vi "Save Station Information.vi"(8 "error in (no error)":errorcluster, 10 "Station Info":T1, 11 "csv-formatter in":refnum<class "csv-formatter.lvclass">) -> (0 "error out":errorcluster, 3 "csv-formatter out":refnum<class "csv-formatter.lvclass">)   [LabVIEW 2015, in "csv-formatter.lvclass"]
doc: "This VI will save the DUT Information to the permanent report"
uses:
  csv-formatter.lvclass
  Report Information/Station Information.ctl
  csv-formatter.lvclass/csv-formatter.ctl
  Report Information/Report Information.lvclass
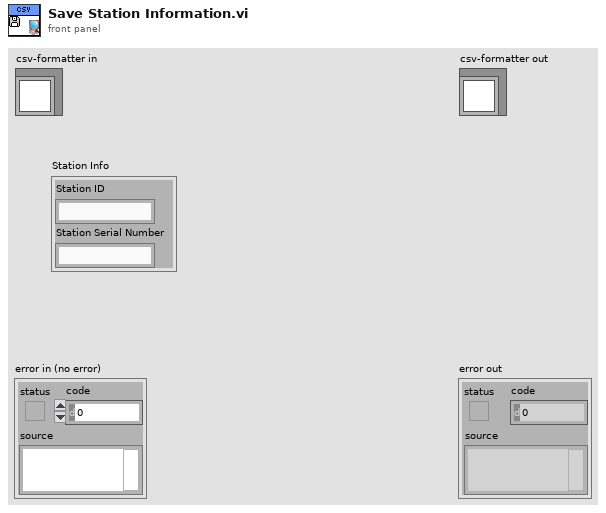
[diagram p1: front panel]
types:
  T1 = typedef "Report Information.lvclass/Station Information.ctl" = cluster{"Station ID":string, "Station Serial Number":string}
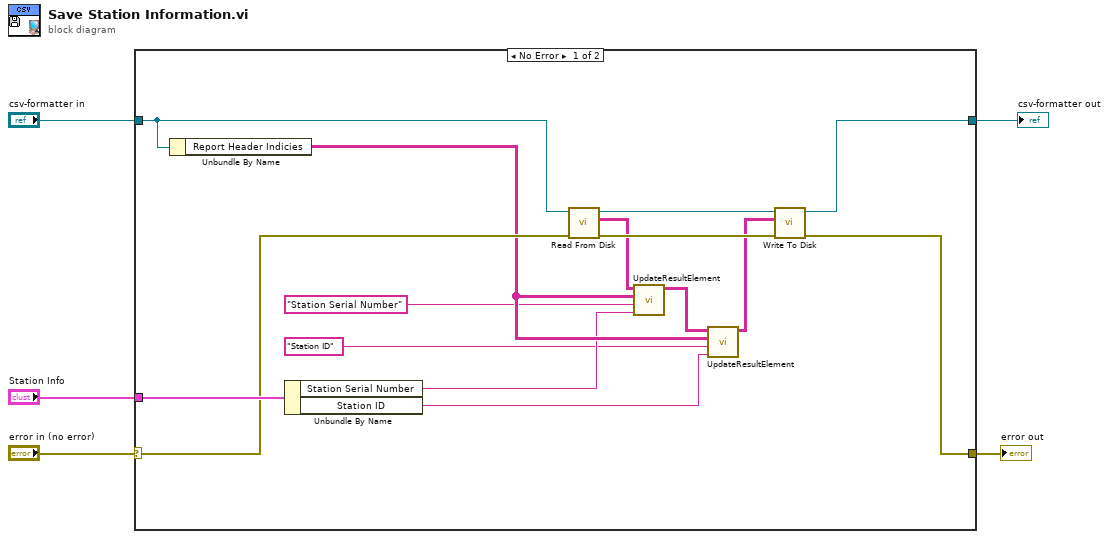
[diagram p0: block diagram]
diagram:
  n1 = case shown="No Error" "error in (no error)" {
    selector: "error in (no error)" -> [w19 w22]
    tunnel: "Station Info" -> [w20 _]
    tunnel: "csv-formatter in" -> [w14 w21]
    tunnel: [w17 w22] -> w2
    tunnel: [w15 w21] -> w1
    frame No Error {
      n2 = Unbundle By Name(w14) -> ("Report Header Indicies"=w10:string[][])
      n3 = Unbundle By Name(w20) -> ("Station Serial Number"=w8:string, "Station ID"=w6:string)
      n4 = call "Read From Disk.vi"("error in (no error)"=w19, "csv-formatter in"=w14) -> ("error out"=w18:errorcluster, "Result Out"=w12:string[][], "csv-formatter out"=w16:refnum<class "csv-formatter.lvclass">)  [unwired: 7 in]
      n5 = call "UpdateResultElement.vi"("Data"=w8, "Lookup String"="Station Serial Number", "Report Header Indicies in"=w10, "Result in"=w12) -> ("Result Out"=w13:string[][])  [unwired: 6 in, 1 out]
      n6 = call "UpdateResultElement.vi"("Data"=w6, "Lookup String"="Station ID", "Report Header Indicies in"=w10, "Result in"=w13) -> ("Result Out"=w11:string[][])  [unwired: 6 in, 1 out]
      n7 = call "Write To Disk.vi"("error in (no error)"=w18, "Result In"=w11, "csv-formatter in"=w16) -> ("error out"=w17:errorcluster, "csv-formatter out"=w15:refnum<class "csv-formatter.lvclass">)  [unwired: 7 in]
    }
    frame Error {
    }
  }
  "error out" <- w2
  "csv-formatter out" <- w1
